vi "AalborgMFC.vi"(7 "Value to Output":dbl format="%.2f", 8 "Ch Description":T1={"Ch Name"="Valve8", "Type"="DLI WebPowerSwitch", "Function"=enum."Relay Output", "Ch State"=enum."On", "Calibration type"="", "A"=200.0, "B"=0.0, "C"=0.0, "D"=0.0, "Comments"="", "Address"={"Main"=0, "Ch."=1, "Sub"=0, "Port Name"="192.168.126.155"}, "String"="LV:LV", "Duty"=65535} {"Duty" format="%016b"; "D" format="%#_5g"; "C" format="%#_5g"; "B" format="%#_5g"; "A" format="%#_5g"}) -> (0 "Scan comment":string, 1 "Output":dbl format="%.3f", 3 "HelpText":string="Value to Output: 1-On 0-Off 99-Toggle\nOutput state is read back, and will be 0 for Off, 1 for On\n\"Port Name\" contains the IP address of the unit\nCh. is used to specify the outlet number, 1-8\nComment (the red box) is used for username:password\n\"A\" is the timeout, in ms")   [LabVIEW 2016]
uses:
  ADAM Client/Sub VIs/ADAM Controls/Ch_description_ADAM.ctl
  ADAM Client/Sub VIs/ADAM Controls/Module_type_ADAM.ctl
  ADAM Client/Sub VIs/ADAM Controls/Function_ADAM.ctl
  ADAM Client/Sub VIs/ADAM Controls/Channel_State.ctl
  ADAM Client/Sub VIs/ADAM Controls/Calib_type_ADAM.ctl
  ADAM Client/Sub VIs/ADAM Controls/Address.ctl
  subVIs/AalborgDFCCommand.ctl
panel:
  out "GoodComms":bool
  # "VI to control Aalborg Digital Mass Flow Controller"
  # "https://www.aalborg.com/index.php/main_page/product_overview/id_product_overview/24"
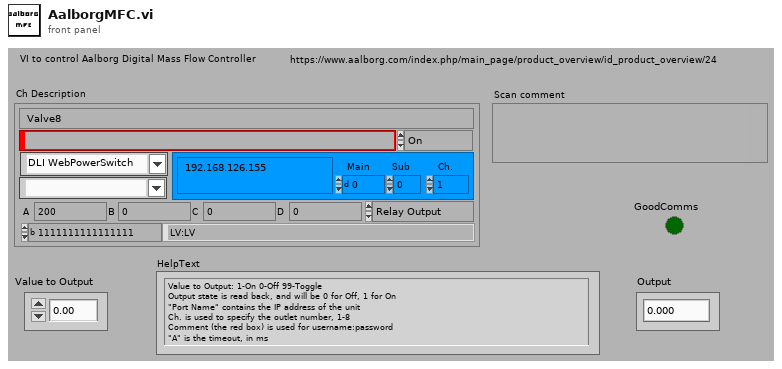
[diagram p1: front panel]
types:
  T1 = typedef "Ch_description_ADAM.ctl" = cluster{"Ch Name":string, "Type":T2, "Function":T3, "Ch State":T4, "Calibration type":T5, "A":dbl, "B":dbl, "C":dbl, "D":dbl, "Comments":string, "Address":T6, "String":string, "Duty":u16}
  T2 = typedef "Module_type_ADAM.ctl" = string
  T3 = typedef "Function_ADAM.ctl" = enum16{"Analogue Input", "Digital Input", "Event counter", "Event rate", "Analogue Output", "Digital Output", "Relay Output"}
  T4 = typedef "Channel_State.ctl" = enum16{"On", "Off", "Always On", "Always Off"}
  T5 = typedef "Calib_type_ADAM.ctl" = string
  T6 = typedef "Address.ctl" = cluster{"Main":i32, "Ch.":i32, "Sub":i32, "Port Name":string}
  T7 = typedef "AalborgDFCCommand.ctl" = string
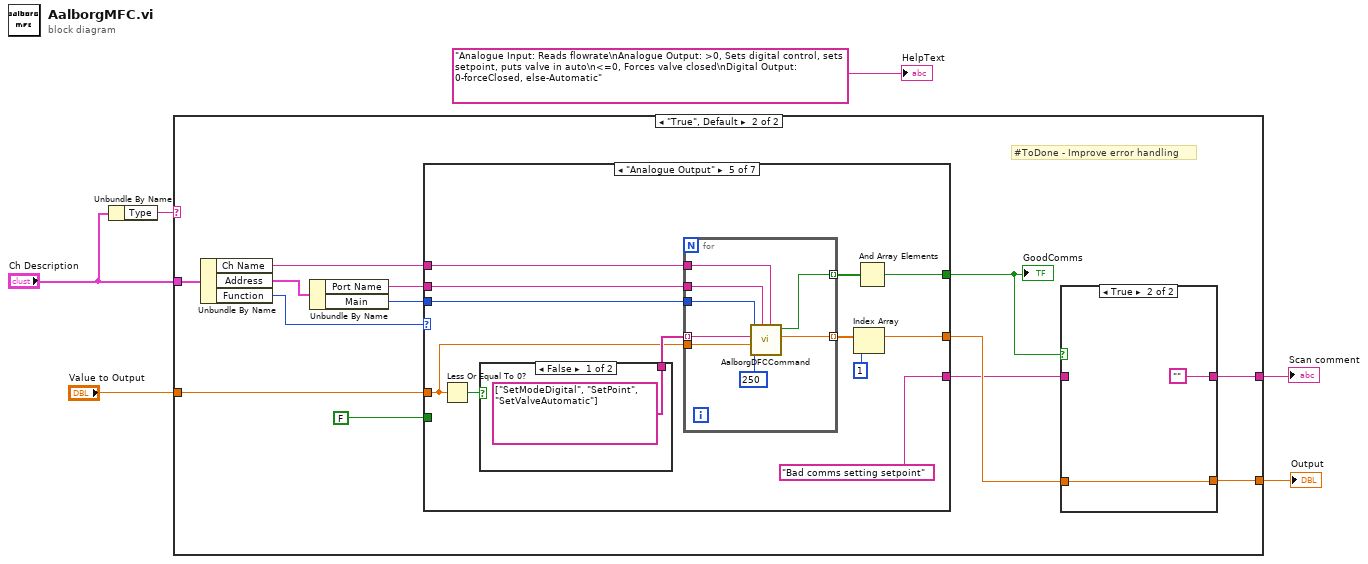
[diagram p0: block diagram]
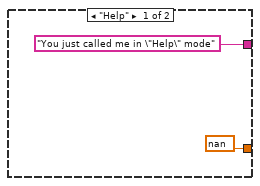
[diagram p2: hidden frame]
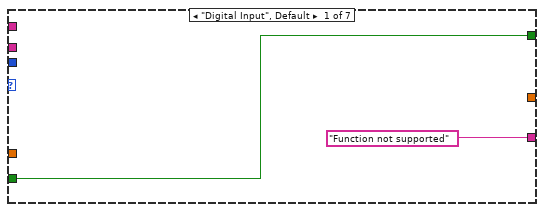
[diagram p3: hidden frame]
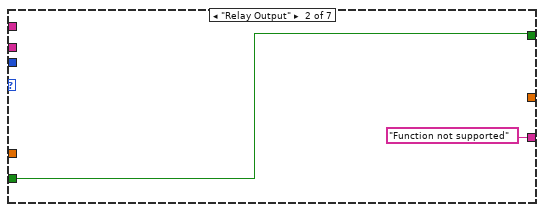
[diagram p4: hidden frame]
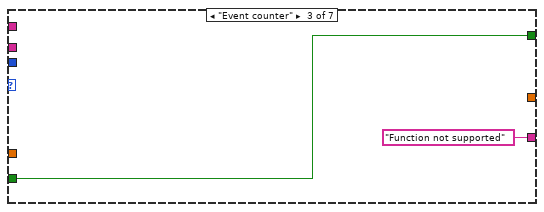
[diagram p5: hidden frame]
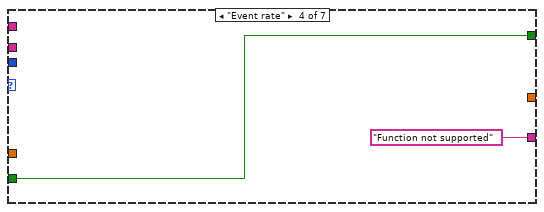
[diagram p6: hidden frame]
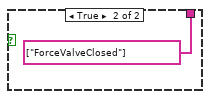
[diagram p7: hidden frame]
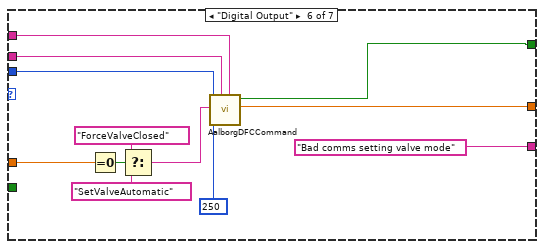
[diagram p8: hidden frame]
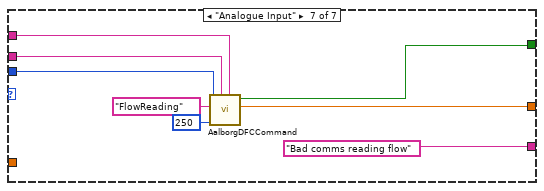
[diagram p9: hidden frame]
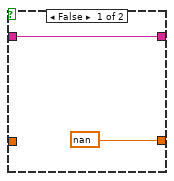
[diagram p10: hidden frame]
diagram:
  n1 = Unbundle By Name("Ch Description") -> ("Type"=w3:T2)
  n2 = case shown="\"True\", Default" w3 {
    tunnel: ["You just called me in \"Help\" mode" w20] -> w6
    tunnel: [nan ("t") w19] -> w5
    tunnel: "Ch Description" -> [_ w17]
    tunnel: "Value to Output" -> [_ w12]
    frame "Help" {
    }
    frame "True", Default {
      # "#ToDone - Improve error handling"
      n3 = Unbundle By Name(w17) -> ("Ch Name"=w13:string, "Address"=w21:T6, "Function"=w16:T3)
      n4 = Unbundle By Name(w21) -> ("Port Name"=w15:string, "Main"=w18:i32)
      n5 = case shown="\"Analogue Output\"" w16 {
        tunnel: w18 -> [_ _ _ _ w40 w62 w70]
        tunnel: w15 -> [_ _ _ _ w41 w63 w71]
        tunnel: [_ _ _ _ w34 w61 w68] -> w14
        tunnel: w13 -> [_ _ _ _ w39 w60 w67]
        tunnel: w12 -> [_ _ _ _ w36 w59 _]
        tunnel: [w23 w25 w27 w29 w31 w54 w66] -> w11
        tunnel: FALSE -> [w23 w25 w27 w29 _ _ _]
        tunnel: ["Function not supported" "Function not supported" "Function not supported" "Function not supported" "Bad comms setting setpoint" "Bad comms setting valve mode" "Bad comms reading flow"] -> w9
        frame "Digital Input", Default {
        }
        frame "Relay Output" {
        }
        frame "Event counter" {
        }
        frame "Event rate" {
        }
        frame "Analogue Output" {
          n6 = Less Or Equal To 0?(x=w36) -> (x <= 0?=w35:bool)
          n7 = case shown="False" w35 {
            tunnel: [T7[] ["SetModeDigital", "SetPoint", "SetValveAutomatic"] T7[] ["ForceValveClosed"]] -> w37
            frame False {
            }
            frame True {
            }
          }
          n8 = for {
            tunnel: w41 -> [w51]
            tunnel: w40 -> [w50]
            tunnel: w37 -> [w49] mode=indexing
            tunnel: w39 -> [w48]
            tunnel: w36 -> [w46]
            tunnel: [w45] -> w38 mode=indexing
            tunnel: [w44] -> w32 mode=indexing
            n9 = call "AalborgDFCCommand.vi"("Channel Name"=w48, "Port Name"=w51, "Timeout/ms"=u32 250, "Numeric Value"=w46, "AalborgDFCCommand"=w49, "Address"=w50) -> ("Numeric Reply"=w45:dbl, "OK"=w44:bool)  [unwired: 1 in, 2 out]
          }
          n10 = Index Array(array=w38, index=1) -> (element=w34:dbl)
          n11 = And Array Elements(Boolean array=w32) -> (logical AND=w31:bool)
        }
        frame "Digital Output" {
          n12 = Equal To 0?(x=w59) -> (x = 0?=w58:bool)
          n13 = Select(t=T7 "ForceValveClosed" ("AalborgDFCCommand"), s=w58, f=T7 "SetValveAutomatic" ("AalborgDFCCommand")) -> (s? t:f=w55:T7)
          n14 = call "AalborgDFCCommand.vi"("Channel Name"=w60, "Port Name"=w63, "Timeout/ms"=u32 250, "AalborgDFCCommand"=w55, "Address"=w62) -> ("Numeric Reply"=w61:dbl, "OK"=w54:bool)  [unwired: 2 in, 2 out]
        }
        frame "Analogue Input" {
          n15 = call "AalborgDFCCommand.vi"("Channel Name"=w67, "Port Name"=w71, "Timeout/ms"=u32 250, "AalborgDFCCommand"=T7 "FlowReading", "Address"=w70) -> ("Numeric Reply"=w68:dbl, "OK"=w66:bool)  [unwired: 2 in, 2 out]
        }
      }
      "GoodComms" <- w11
      n16 = case shown="True" w11 {
        tunnel: [w72 ""] -> w20
        tunnel: [nan ("t") w74] -> w19
        tunnel: w14 -> [_ w74]
        tunnel: w9 -> [w72 _]
        frame False {
        }
        frame True {
        }
      }
    }
  }
  "Output" <- w5
  "Scan comment" <- w6
  "HelpText" <- "Analogue Input: Reads flowrate\nAnalogue Output: >0, Sets digital control, sets setpoint, puts valve in auto\n<=0, Forces valve closed\nDigital Output: 0-forceClosed, else-Automatic"
